vi "Read Gas Ref.vi"(8 "error in (no error)":errorcluster, 11 "Particle Properties in":refnum<class "Particle Properties.lvclass">) -> (0 "error out":errorcluster, 2 "Gas Ref":refnum<data-value>, 3 "Particle Properties out":refnum<class "Particle Properties.lvclass">)   [LabVIEW 2015, in "Particle Properties.lvclass"]
uses:
  Particle Properties.lvclass
  Atmospheric/Gas Properties/Gas Properties.lvclass
  Particle Properties.lvclass/Particle Properties.ctl
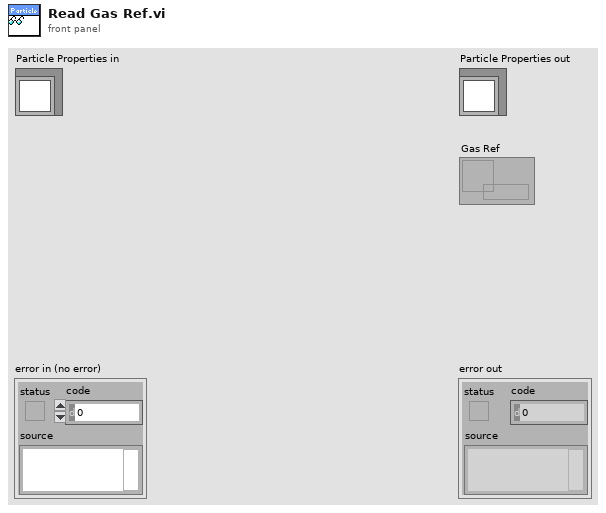
[diagram p1: front panel]
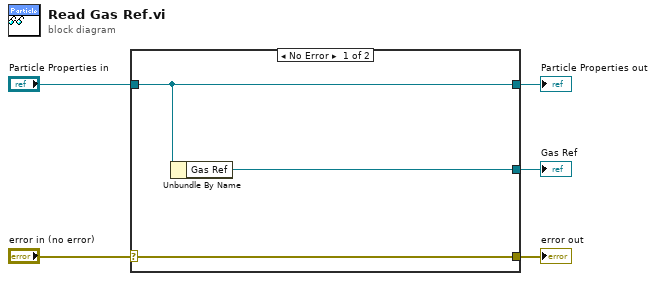
[diagram p0: block diagram]
diagram:
  n1 = case shown="No Error" "error in (no error)" {
    selector: "error in (no error)" -> [w8 w9]
    tunnel: [w8 w9] -> w4
    tunnel: [w7 w10] -> w2
    tunnel: "Particle Properties in" -> [w7 w10]
    tunnel: [w6 _] -> w1
    frame No Error {
      n2 = Unbundle By Name(w7) -> ("Gas Ref"=w6:refnum<data-value>)
    }
    frame Error {
    }
  }
  "error out" <- w4
  "Particle Properties out" <- w2
  "Gas Ref" <- w1
